vi "create config for small chassi.vi"() -> ()   [LabVIEW 2020]
uses:
  <instrlib>/_niInstr/Data Trigger/v1/Shared/Public/Edge Configuration Trigger Slope.ctl
  <vilib>/Utility/xml.llb/Write to XML File(string).vi
  <instrlib>/_niInstr/Data Trigger/v1/Shared/niInstr Data Trigger v1 Shared.lvlib
panel:
  in  "diff const [ns] 6":dbl
  in  "strob duration[ns] 5":dbl
  in  "Chans enable 6":T1={"Chan 0"=TRUE, "Chan 1"=TRUE, "Chan 2"=FALSE, "Chan 3"=FALSE, "Chan 4"=FALSE, "Chan 5"=FALSE, "Chan 6"=FALSE, "Chan 7"=FALSE}
  in  "Trapez config 6":T2={"k [ns] "=1100, "m [ns] "=200, "t_decay [ns]  "=65000, "Get energy at %\n of flat top"=70}
  in  "common trig 5172":T4={"level (V)"=-0.01, "hysteresis (V)"=0.001, "trigger slope"=enum."Negative"}
  in  "common trig 5170R 2-3":T4={"level (V)"=-0.01, "hysteresis (V)"=0.001, "trigger slope"=enum."Negative"}
  in  "common trig 5170R 0-1":T4={"level (V)"=-0.01, "hysteresis (V)"=0.001, "trigger slope"=enum."Negative"}
  in  "Enum":enum16{"Set common configs", "Write XML file"}(ring)
  in  "file name":string
  out "Writing done successfully":bool
  in  "folder":path
  in  "TAC delay":dbl
  in  "marker duration":dbl
  in  "shift marker":dbl
  in  "f":dbl
  in  "trig cfd":T4={"level (V)"=-0.01, "hysteresis (V)"=0.001, "trigger slope"=enum."Negative"}
  in  "trig marker":T4={"level (V)"=-0.01, "hysteresis (V)"=0.001, "trigger slope"=enum."Negative"}
  in  "diff const [ns] 5":dbl
  in  "BGO marker\nduration[ns] 5":dbl
  in  "Trigger Cluster 5":T5={"trig config 0"={"level (V)"=-0.01, "hysteresis (V)"=0.001, "trigger slope"=enum."Negative"}, "trig config 1"={"level (V)"=-0.01, "hysteresis (V)"=0.001, "trigger slope"=enum."Negative"}, "trig config 2"={"level (V)"=0.0, "hysteresis (V)"=0.0, "trigger slope"=enum."Positive"}, "trig config 3"={"level (V)"=0.0, "hysteresis (V)"=0.0, "trigger slope"=enum."Positive"}, "trig config 4"={"level (V)"=0.0, "hysteresis (V)"=0.0, "trigger slope"=enum."Positive"}, "trig config 5"={"level (V)"=0.0, "hysteresis (V)"=0.0, "trigger slope"=enum."Positive"}, "trig config 6"={"level (V)"=0.0, "hysteresis (V)"=0.0, "trigger slope"=enum."Positive"}, "trig config 7"={"level (V)"=0.0, "hysteresis (V)"=0.0, "trigger slope"=enum."Positive"}}
  in  "Calibr coef 5":T6={"calibr coef ch 0"={"a"=1.0, "b"=0.0}, "calibr coef ch 1"={"a"=1.0, "b"=0.0}, "calibr coef ch 2"={"a"=1.0, "b"=0.0}, "calibr coef ch 3"={"a"=1.0, "b"=0.0}, "calibr coef ch 4"={"a"=1.0, "b"=0.0}, "calibr coef ch 5"={"a"=1.0, "b"=0.0}, "calibr coef ch 6"={"a"=1.0, "b"=0.0}, "calibr coef ch 7"={"a"=1.0, "b"=0.0}}
  in  "Trapez config 5":T2={"k [ns] "=1100, "m [ns] "=200, "t_decay [ns]  "=65000, "Get energy at %\n of flat top"=70}
  in  "Chans enable 5":T1={"Chan 0"=TRUE, "Chan 1"=TRUE, "Chan 2"=FALSE, "Chan 3"=FALSE, "Chan 4"=FALSE, "Chan 5"=FALSE, "Chan 6"=FALSE, "Chan 7"=FALSE}
  in  "diff const [ns] 4":dbl
  in  "strob duration[ns] 4":dbl
  in  "Trigger Cluster 4":T5={"trig config 0"={"level (V)"=-0.01, "hysteresis (V)"=0.001, "trigger slope"=enum."Negative"}, "trig config 1"={"level (V)"=-0.01, "hysteresis (V)"=0.001, "trigger slope"=enum."Negative"}, "trig config 2"={"level (V)"=0.0, "hysteresis (V)"=0.0, "trigger slope"=enum."Positive"}, "trig config 3"={"level (V)"=0.0, "hysteresis (V)"=0.0, "trigger slope"=enum."Positive"}, "trig config 4"={"level (V)"=0.0, "hysteresis (V)"=0.0, "trigger slope"=enum."Positive"}, "trig config 5"={"level (V)"=0.0, "hysteresis (V)"=0.0, "trigger slope"=enum."Positive"}, "trig config 6"={"level (V)"=0.0, "hysteresis (V)"=0.0, "trigger slope"=enum."Positive"}, "trig config 7"={"level (V)"=0.0, "hysteresis (V)"=0.0, "trigger slope"=enum."Positive"}}
  in  "Calibr coef 4":T6={"calibr coef ch 0"={"a"=1.0, "b"=0.0}, "calibr coef ch 1"={"a"=1.0, "b"=0.0}, "calibr coef ch 2"={"a"=1.0, "b"=0.0}, "calibr coef ch 3"={"a"=1.0, "b"=0.0}, "calibr coef ch 4"={"a"=1.0, "b"=0.0}, "calibr coef ch 5"={"a"=1.0, "b"=0.0}, "calibr coef ch 6"={"a"=1.0, "b"=0.0}, "calibr coef ch 7"={"a"=1.0, "b"=0.0}}
  in  "Trapez config 4":T2={"k [ns] "=1100, "m [ns] "=200, "t_decay [ns]  "=65000, "Get energy at %\n of flat top"=70}
  in  "Chans enable 4":T1={"Chan 0"=TRUE, "Chan 1"=TRUE, "Chan 2"=FALSE, "Chan 3"=FALSE, "Chan 4"=FALSE, "Chan 5"=FALSE, "Chan 6"=FALSE, "Chan 7"=FALSE}
  in  "diff const [ns] 3":dbl
  in  "strob duration[ns] 3":dbl
  in  "Trigger Cluster 3":T5={"trig config 0"={"level (V)"=-0.01, "hysteresis (V)"=0.001, "trigger slope"=enum."Negative"}, "trig config 1"={"level (V)"=-0.01, "hysteresis (V)"=0.001, "trigger slope"=enum."Negative"}, "trig config 2"={"level (V)"=0.0, "hysteresis (V)"=0.0, "trigger slope"=enum."Positive"}, "trig config 3"={"level (V)"=0.0, "hysteresis (V)"=0.0, "trigger slope"=enum."Positive"}, "trig config 4"={"level (V)"=0.0, "hysteresis (V)"=0.0, "trigger slope"=enum."Positive"}, "trig config 5"={"level (V)"=0.0, "hysteresis (V)"=0.0, "trigger slope"=enum."Positive"}, "trig config 6"={"level (V)"=0.0, "hysteresis (V)"=0.0, "trigger slope"=enum."Positive"}, "trig config 7"={"level (V)"=0.0, "hysteresis (V)"=0.0, "trigger slope"=enum."Positive"}}
  in  "Calibr coef 3":T6={"calibr coef ch 0"={"a"=1.0, "b"=0.0}, "calibr coef ch 1"={"a"=1.0, "b"=0.0}, "calibr coef ch 2"={"a"=1.0, "b"=0.0}, "calibr coef ch 3"={"a"=1.0, "b"=0.0}, "calibr coef ch 4"={"a"=1.0, "b"=0.0}, "calibr coef ch 5"={"a"=1.0, "b"=0.0}, "calibr coef ch 6"={"a"=1.0, "b"=0.0}, "calibr coef ch 7"={"a"=1.0, "b"=0.0}}
  in  "Trapez config 3":T2={"k [ns] "=1100, "m [ns] "=200, "t_decay [ns]  "=65000, "Get energy at %\n of flat top"=70}
  in  "Chans enable 3":T1={"Chan 0"=TRUE, "Chan 1"=TRUE, "Chan 2"=FALSE, "Chan 3"=FALSE, "Chan 4"=FALSE, "Chan 5"=FALSE, "Chan 6"=FALSE, "Chan 7"=FALSE}
  in  "diff const [ns] 2":dbl
  in  "strob duration[ns] 2":dbl
  in  "Trigger Cluster 2":T5={"trig config 0"={"level (V)"=-0.01, "hysteresis (V)"=0.001, "trigger slope"=enum."Negative"}, "trig config 1"={"level (V)"=-0.01, "hysteresis (V)"=0.001, "trigger slope"=enum."Negative"}, "trig config 2"={"level (V)"=0.0, "hysteresis (V)"=0.0, "trigger slope"=enum."Positive"}, "trig config 3"={"level (V)"=0.0, "hysteresis (V)"=0.0, "trigger slope"=enum."Positive"}, "trig config 4"={"level (V)"=0.0, "hysteresis (V)"=0.0, "trigger slope"=enum."Positive"}, "trig config 5"={"level (V)"=0.0, "hysteresis (V)"=0.0, "trigger slope"=enum."Positive"}, "trig config 6"={"level (V)"=0.0, "hysteresis (V)"=0.0, "trigger slope"=enum."Positive"}, "trig config 7"={"level (V)"=0.0, "hysteresis (V)"=0.0, "trigger slope"=enum."Positive"}}
  in  "Calibr coef 2":T6={"calibr coef ch 0"={"a"=1.0, "b"=0.0}, "calibr coef ch 1"={"a"=1.0, "b"=0.0}, "calibr coef ch 2"={"a"=1.0, "b"=0.0}, "calibr coef ch 3"={"a"=1.0, "b"=0.0}, "calibr coef ch 4"={"a"=1.0, "b"=0.0}, "calibr coef ch 5"={"a"=1.0, "b"=0.0}, "calibr coef ch 6"={"a"=1.0, "b"=0.0}, "calibr coef ch 7"={"a"=1.0, "b"=0.0}}
  in  "Trapez config 2":T2={"k [ns] "=1100, "m [ns] "=200, "t_decay [ns]  "=65000, "Get energy at %\n of flat top"=70}
  in  "Chans enable 2":T1={"Chan 0"=TRUE, "Chan 1"=TRUE, "Chan 2"=FALSE, "Chan 3"=FALSE, "Chan 4"=FALSE, "Chan 5"=FALSE, "Chan 6"=FALSE, "Chan 7"=FALSE}
  in  "diff const [ns]":dbl
  in  "strob duration[ns]":dbl
  in  "Trigger Cluster":T5={"trig config 0"={"level (V)"=-0.01, "hysteresis (V)"=0.001, "trigger slope"=enum."Negative"}, "trig config 1"={"level (V)"=-0.01, "hysteresis (V)"=0.001, "trigger slope"=enum."Negative"}, "trig config 2"={"level (V)"=0.0, "hysteresis (V)"=0.0, "trigger slope"=enum."Positive"}, "trig config 3"={"level (V)"=0.0, "hysteresis (V)"=0.0, "trigger slope"=enum."Positive"}, "trig config 4"={"level (V)"=0.0, "hysteresis (V)"=0.0, "trigger slope"=enum."Positive"}, "trig config 5"={"level (V)"=0.0, "hysteresis (V)"=0.0, "trigger slope"=enum."Positive"}, "trig config 6"={"level (V)"=0.0, "hysteresis (V)"=0.0, "trigger slope"=enum."Positive"}, "trig config 7"={"level (V)"=0.0, "hysteresis (V)"=0.0, "trigger slope"=enum."Positive"}}
  in  "Calibr coef":T6={"calibr coef ch 0"={"a"=1.0, "b"=0.0}, "calibr coef ch 1"={"a"=1.0, "b"=0.0}, "calibr coef ch 2"={"a"=1.0, "b"=0.0}, "calibr coef ch 3"={"a"=1.0, "b"=0.0}, "calibr coef ch 4"={"a"=1.0, "b"=0.0}, "calibr coef ch 5"={"a"=1.0, "b"=0.0}, "calibr coef ch 6"={"a"=1.0, "b"=0.0}, "calibr coef ch 7"={"a"=1.0, "b"=0.0}}
  in  "Trapez config":T2={"k [ns] "=1100, "m [ns] "=200, "t_decay [ns]  "=65000, "Get energy at %\n of flat top"=70}
  in  "Chans enable":T1={"Chan 0"=TRUE, "Chan 1"=TRUE, "Chan 2"=FALSE, "Chan 3"=FALSE, "Chan 4"=FALSE, "Chan 5"=FALSE, "Chan 6"=FALSE, "Chan 7"=FALSE}
  # "PXIe 5170R 0"
  # "PXIe 5170R 1"
  # "PXIe 5170R 2"
  # "PXIe 5170R 3"
  # "PXIe 5172 [clover]"
  # "PXIe 5764"
  # "common configs"
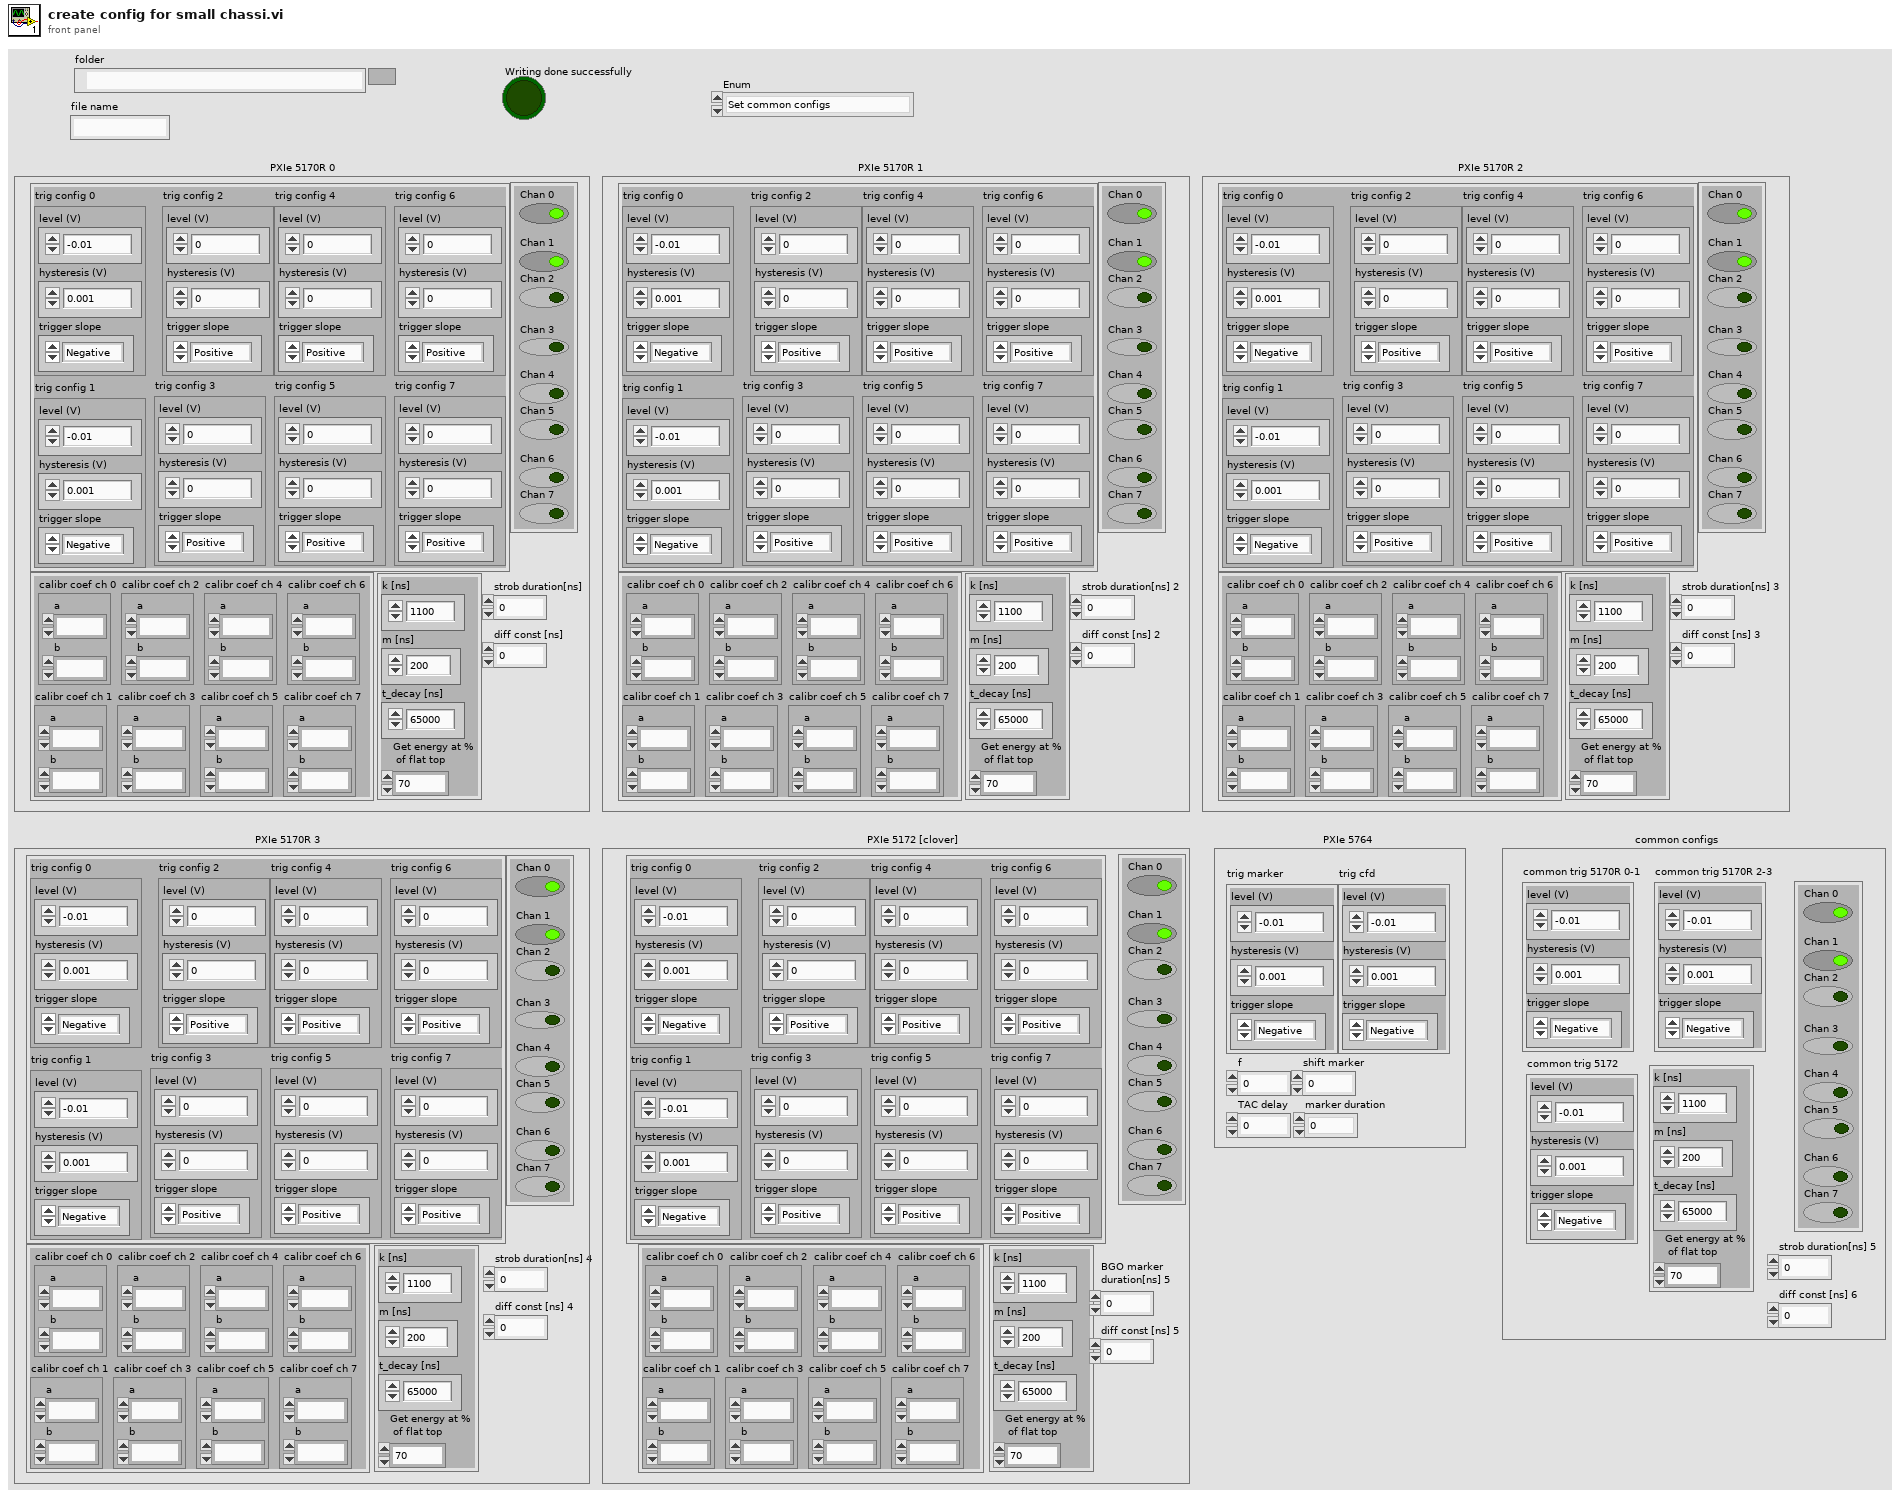
[diagram p1: front panel]
types:
  T1 = cluster{"Chan 0":bool, "Chan 1":bool, "Chan 2":bool, "Chan 3":bool, "Chan 4":bool, "Chan 5":bool, "Chan 6":bool, "Chan 7":bool}
  T2 = cluster{"k [ns] ":u16, "m [ns] ":u16, "t_decay [ns]  ":u32, "Get energy at %\n of flat top":i8}
  T3 = typedef "niInstr Data Trigger v1 Shared.lvlib/Edge Configuration Trigger Slope.ctl" = enum8{"Positive", "Negative"}
  T4 = cluster{"level (V)":dbl, "hysteresis (V)":dbl, "trigger slope":T3}
  T5 = cluster{"trig config 0":cluster{"level (V)":dbl, "hysteresis (V)":dbl, "trigger slope":T3}, "trig config 1":cluster{"level (V)":dbl, "hysteresis (V)":dbl, "trigger slope":T3}, "trig config 2":cluster{"level (V)":dbl, "hysteresis (V)":dbl, "trigger slope":T3}, "trig config 3":cluster{"level (V)":dbl, "hysteresis (V)":dbl, "trigger slope":T3}, "trig config 4":cluster{"level (V)":dbl, "hysteresis (V)":dbl, "trigger slope":T3}, "trig config 5":cluster{"level (V)":dbl, "hysteresis (V)":dbl, "trigger slope":T3}, "trig config 6":cluster{"level (V)":dbl, "hysteresis (V)":dbl, "trigger slope":T3}, "trig config 7":cluster{"level (V)":dbl, "hysteresis (V)":dbl, "trigger slope":T3}}
  T6 = cluster{"calibr coef ch 0":cluster{"a":fxp<+/-,18,9>, "b":fxp<+/-,48,24>}, "calibr coef ch 1":cluster{"a":fxp<+/-,18,9>, "b":fxp<+/-,48,24>}, "calibr coef ch 2":cluster{"a":fxp<+/-,18,9>, "b":fxp<+/-,48,24>}, "calibr coef ch 3":cluster{"a":fxp<+/-,18,9>, "b":fxp<+/-,48,24>}, "calibr coef ch 4":cluster{"a":fxp<+/-,18,9>, "b":fxp<+/-,48,24>}, "calibr coef ch 5":cluster{"a":fxp<+/-,18,9>, "b":fxp<+/-,48,24>}, "calibr coef ch 6":cluster{"a":fxp<+/-,18,9>, "b":fxp<+/-,48,24>}, "calibr coef ch 7":cluster{"a":fxp<+/-,18,9>, "b":fxp<+/-,48,24>}}
  T7 = cluster{"trig marker":cluster{"level (V)":dbl, "hysteresis (V)":dbl, "trigger slope":T3}, "trig cfd":cluster{"level (V)":dbl, "hysteresis (V)":dbl, "trigger slope":T3}, "f":dbl, "shift marker":dbl, "marker duration":dbl, "TAC delay":dbl}
  T8 = cluster{"Chans enable 5":cluster{"Chan 0":bool, "Chan 1":bool, "Chan 2":bool, "Chan 3":bool, "Chan 4":bool, "Chan 5":bool, "Chan 6":bool, "Chan 7":bool}, "Trapez config 5":cluster{"k [ns] ":u16, "m [ns] ":u16, "t_decay [ns]  ":u32, "Get energy at %\n of flat top":i8}, "Trigger Cluster 5":cluster{"trig config 0":cluster{"level (V)":dbl, "hysteresis (V)":dbl, "trigger slope":T3}, "trig config 1":cluster{"level (V)":dbl, "hysteresis (V)":dbl, "trigger slope":T3}, "trig config 2":cluster{"level (V)":dbl, "hysteresis (V)":dbl, "trigger slope":T3}, "trig config 3":cluster{"level (V)":dbl, "hysteresis (V)":dbl, "trigger slope":T3}, "trig config 4":cluster{"level (V)":dbl, "hysteresis (V)":dbl, "trigger slope":T3}, "trig config 5":cluster{"level (V)":dbl, "hysteresis (V)":dbl, "trigger slope":T3}, "trig config 6":cluster{"level (V)":dbl, "hysteresis (V)":dbl, "trigger slope":T3}, "trig config 7":cluster{"level (V)":dbl, "hysteresis (V)":dbl, "trigger slope":T3}}, "Calibr coef 5":cluster{"calibr coef ch 0":cluster{"a":fxp<+/-,18,9>, "b":fxp<+/-,48,24>}, "calibr coef ch 1":cluster{"a":fxp<+/-,18,9>, "b":fxp<+/-,48,24>}, "calibr coef ch 2":cluster{"a":fxp<+/-,18,9>, "b":fxp<+/-,48,24>}, "calibr coef ch 3":cluster{"a":fxp<+/-,18,9>, "b":fxp<+/-,48,24>}, "calibr coef ch 4":cluster{"a":fxp<+/-,18,9>, "b":fxp<+/-,48,24>}, "calibr coef ch 5":cluster{"a":fxp<+/-,18,9>, "b":fxp<+/-,48,24>}, "calibr coef ch 6":cluster{"a":fxp<+/-,18,9>, "b":fxp<+/-,48,24>}, "calibr coef ch 7":cluster{"a":fxp<+/-,18,9>, "b":fxp<+/-,48,24>}}, "BGO marker\nduration[ns] 5":dbl, "diff const [ns] 5":dbl}
  T9 = cluster{"5170R 0":cluster{"Chans enable":cluster{"Chan 0":bool, "Chan 1":bool, "Chan 2":bool, "Chan 3":bool, "Chan 4":bool, "Chan 5":bool, "Chan 6":bool, "Chan 7":bool}, "Trapez config":cluster{"k [ns] ":u16, "m [ns] ":u16, "t_decay [ns]  ":u32, "Get energy at %\n of flat top":i8}, "Trigger Cluster":cluster{"trig config 0":cluster{"level (V)":dbl, "hysteresis (V)":dbl, "trigger slope":T3}, "trig config 1":cluster{"level (V)":dbl, "hysteresis (V)":dbl, "trigger slope":T3}, "trig config 2":cluster{"level (V)":dbl, "hysteresis (V)":dbl, "trigger slope":T3}, "trig config 3":cluster{"level (V)":dbl, "hysteresis (V)":dbl, "trigger slope":T3}, "trig config 4":cluster{"level (V)":dbl, "hysteresis (V)":dbl, "trigger slope":T3}, "trig config 5":cluster{"level (V)":dbl, "hysteresis (V)":dbl, "trigger slope":T3}, "trig config 6":cluster{"level (V)":dbl, "hysteresis (V)":dbl, "trigger slope":T3}, "trig config 7":cluster{"level (V)":dbl, "hysteresis (V)":dbl, "trigger slope":T3}}, "Calibr coef":cluster{"calibr coef ch 0":cluster{"a":fxp<+/-,18,9>, "b":fxp<+/-,48,24>}, "calibr coef ch 1":cluster{"a":fxp<+/-,18,9>, "b":fxp<+/-,48,24>}, "calibr coef ch 2":cluster{"a":fxp<+/-,18,9>, "b":fxp<+/-,48,24>}, "calibr coef ch 3":cluster{"a":fxp<+/-,18,9>, "b":fxp<+/-,48,24>}, "calibr coef ch 4":cluster{"a":fxp<+/-,18,9>, "b":fxp<+/-,48,24>}, "calibr coef ch 5":cluster{"a":fxp<+/-,18,9>, "b":fxp<+/-,48,24>}, "calibr coef ch 6":cluster{"a":fxp<+/-,18,9>, "b":fxp<+/-,48,24>}, "calibr coef ch 7":cluster{"a":fxp<+/-,18,9>, "b":fxp<+/-,48,24>}}, "strob duration[ns]":dbl, "diff const [ns]":dbl}, "5170R 1":cluster{"Chans enable":cluster{"Chan 0":bool, "Chan 1":bool, "Chan 2":bool, "Chan 3":bool, "Chan 4":bool, "Chan 5":bool, "Chan 6":bool, "Chan 7":bool}, "Trapez config":cluster{"k [ns] ":u16, "m [ns] ":u16, "t_decay [ns]  ":u32, "Get energy at %\n of flat top":i8}, "Trigger Cluster":cluster{"trig config 0":cluster{"level (V)":dbl, "hysteresis (V)":dbl, "trigger slope":T3}, "trig config 1":cluster{"level (V)":dbl, "hysteresis (V)":dbl, "trigger slope":T3}, "trig config 2":cluster{"level (V)":dbl, "hysteresis (V)":dbl, "trigger slope":T3}, "trig config 3":cluster{"level (V)":dbl, "hysteresis (V)":dbl, "trigger slope":T3}, "trig config 4":cluster{"level (V)":dbl, "hysteresis (V)":dbl, "trigger slope":T3}, "trig config 5":cluster{"level (V)":dbl, "hysteresis (V)":dbl, "trigger slope":T3}, "trig config 6":cluster{"level (V)":dbl, "hysteresis (V)":dbl, "trigger slope":T3}, "trig config 7":cluster{"level (V)":dbl, "hysteresis (V)":dbl, "trigger slope":T3}}, "Calibr coef":cluster{"calibr coef ch 0":cluster{"a":fxp<+/-,18,9>, "b":fxp<+/-,48,24>}, "calibr coef ch 1":cluster{"a":fxp<+/-,18,9>, "b":fxp<+/-,48,24>}, "calibr coef ch 2":cluster{"a":fxp<+/-,18,9>, "b":fxp<+/-,48,24>}, "calibr coef ch 3":cluster{"a":fxp<+/-,18,9>, "b":fxp<+/-,48,24>}, "calibr coef ch 4":cluster{"a":fxp<+/-,18,9>, "b":fxp<+/-,48,24>}, "calibr coef ch 5":cluster{"a":fxp<+/-,18,9>, "b":fxp<+/-,48,24>}, "calibr coef ch 6":cluster{"a":fxp<+/-,18,9>, "b":fxp<+/-,48,24>}, "calibr coef ch 7":cluster{"a":fxp<+/-,18,9>, "b":fxp<+/-,48,24>}}, "strob duration[ns]":dbl, "diff const [ns]":dbl}, "5170R 2":cluster{"Chans enable":cluster{"Chan 0":bool, "Chan 1":bool, "Chan 2":bool, "Chan 3":bool, "Chan 4":bool, "Chan 5":bool, "Chan 6":bool, "Chan 7":bool}, "Trapez config":cluster{"k [ns] ":u16, "m [ns] ":u16, "t_decay [ns]  ":u32, "Get energy at %\n of flat top":i8}, "Trigger Cluster":cluster{"trig config 0":cluster{"level (V)":dbl, "hysteresis (V)":dbl, "trigger slope":T3}, "trig config 1":cluster{"level (V)":dbl, "hysteresis (V)":dbl, "trigger slope":T3}, "trig config 2":cluster{"level (V)":dbl, "hysteresis (V)":dbl, "trigger slope":T3}, "trig config 3":cluster{"level (V)":dbl, "hysteresis (V)":dbl, "trigger slope":T3}, "trig config 4":cluster{"level (V)":dbl, "hysteresis (V)":dbl, "trigger slope":T3}, "trig config 5":cluster{"level (V)":dbl, "hysteresis (V)":dbl, "trigger slope":T3}, "trig config 6":cluster{"level (V)":dbl, "hysteresis (V)":dbl, "trigger slope":T3}, "trig config 7":cluster{"level (V)":dbl, "hysteresis (V)":dbl, "trigger slope":T3}}, "Calibr coef":cluster{"calibr coef ch 0":cluster{"a":fxp<+/-,18,9>, "b":fxp<+/-,48,24>}, "calibr coef ch 1":cluster{"a":fxp<+/-,18,9>, "b":fxp<+/-,48,24>}, "calibr coef ch 2":cluster{"a":fxp<+/-,18,9>, "b":fxp<+/-,48,24>}, "calibr coef ch 3":cluster{"a":fxp<+/-,18,9>, "b":fxp<+/-,48,24>}, "calibr coef ch 4":cluster{"a":fxp<+/-,18,9>, "b":fxp<+/-,48,24>}, "calibr coef ch 5":cluster{"a":fxp<+/-,18,9>, "b":fxp<+/-,48,24>}, "calibr coef ch 6":cluster{"a":fxp<+/-,18,9>, "b":fxp<+/-,48,24>}, "calibr coef ch 7":cluster{"a":fxp<+/-,18,9>, "b":fxp<+/-,48,24>}}, "strob duration[ns]":dbl, "diff const [ns]":dbl}, "5170R 3":cluster{"Chans enable":cluster{"Chan 0":bool, "Chan 1":bool, "Chan 2":bool, "Chan 3":bool, "Chan 4":bool, "Chan 5":bool, "Chan 6":bool, "Chan 7":bool}, "Trapez config":cluster{"k [ns] ":u16, "m [ns] ":u16, "t_decay [ns]  ":u32, "Get energy at %\n of flat top":i8}, "Trigger Cluster":cluster{"trig config 0":cluster{"level (V)":dbl, "hysteresis (V)":dbl, "trigger slope":T3}, "trig config 1":cluster{"level (V)":dbl, "hysteresis (V)":dbl, "trigger slope":T3}, "trig config 2":cluster{"level (V)":dbl, "hysteresis (V)":dbl, "trigger slope":T3}, "trig config 3":cluster{"level (V)":dbl, "hysteresis (V)":dbl, "trigger slope":T3}, "trig config 4":cluster{"level (V)":dbl, "hysteresis (V)":dbl, "trigger slope":T3}, "trig config 5":cluster{"level (V)":dbl, "hysteresis (V)":dbl, "trigger slope":T3}, "trig config 6":cluster{"level (V)":dbl, "hysteresis (V)":dbl, "trigger slope":T3}, "trig config 7":cluster{"level (V)":dbl, "hysteresis (V)":dbl, "trigger slope":T3}}, "Calibr coef":cluster{"calibr coef ch 0":cluster{"a":fxp<+/-,18,9>, "b":fxp<+/-,48,24>}, "calibr coef ch 1":cluster{"a":fxp<+/-,18,9>, "b":fxp<+/-,48,24>}, "calibr coef ch 2":cluster{"a":fxp<+/-,18,9>, "b":fxp<+/-,48,24>}, "calibr coef ch 3":cluster{"a":fxp<+/-,18,9>, "b":fxp<+/-,48,24>}, "calibr coef ch 4":cluster{"a":fxp<+/-,18,9>, "b":fxp<+/-,48,24>}, "calibr coef ch 5":cluster{"a":fxp<+/-,18,9>, "b":fxp<+/-,48,24>}, "calibr coef ch 6":cluster{"a":fxp<+/-,18,9>, "b":fxp<+/-,48,24>}, "calibr coef ch 7":cluster{"a":fxp<+/-,18,9>, "b":fxp<+/-,48,24>}}, "strob duration[ns]":dbl, "diff const [ns]":dbl}, "5172":cluster{"Chans enable 5":cluster{"Chan 0":bool, "Chan 1":bool, "Chan 2":bool, "Chan 3":bool, "Chan 4":bool, "Chan 5":bool, "Chan 6":bool, "Chan 7":bool}, "Trapez config 5":cluster{"k [ns] ":u16, "m [ns] ":u16, "t_decay [ns]  ":u32, "Get energy at %\n of flat top":i8}, "Trigger Cluster 5":cluster{"trig config 0":cluster{"level (V)":dbl, "hysteresis (V)":dbl, "trigger slope":T3}, "trig config 1":cluster{"level (V)":dbl, "hysteresis (V)":dbl, "trigger slope":T3}, "trig config 2":cluster{"level (V)":dbl, "hysteresis (V)":dbl, "trigger slope":T3}, "trig config 3":cluster{"level (V)":dbl, "hysteresis (V)":dbl, "trigger slope":T3}, "trig config 4":cluster{"level (V)":dbl, "hysteresis (V)":dbl, "trigger slope":T3}, "trig config 5":cluster{"level (V)":dbl, "hysteresis (V)":dbl, "trigger slope":T3}, "trig config 6":cluster{"level (V)":dbl, "hysteresis (V)":dbl, "trigger slope":T3}, "trig config 7":cluster{"level (V)":dbl, "hysteresis (V)":dbl, "trigger slope":T3}}, "Calibr coef 5":cluster{"calibr coef ch 0":cluster{"a":fxp<+/-,18,9>, "b":fxp<+/-,48,24>}, "calibr coef ch 1":cluster{"a":fxp<+/-,18,9>, "b":fxp<+/-,48,24>}, "calibr coef ch 2":cluster{"a":fxp<+/-,18,9>, "b":fxp<+/-,48,24>}, "calibr coef ch 3":cluster{"a":fxp<+/-,18,9>, "b":fxp<+/-,48,24>}, "calibr coef ch 4":cluster{"a":fxp<+/-,18,9>, "b":fxp<+/-,48,24>}, "calibr coef ch 5":cluster{"a":fxp<+/-,18,9>, "b":fxp<+/-,48,24>}, "calibr coef ch 6":cluster{"a":fxp<+/-,18,9>, "b":fxp<+/-,48,24>}, "calibr coef ch 7":cluster{"a":fxp<+/-,18,9>, "b":fxp<+/-,48,24>}}, "BGO marker\nduration[ns] 5":dbl, "diff const [ns] 5":dbl}, "5764":cluster{"trig marker":cluster{"level (V)":dbl, "hysteresis (V)":dbl, "trigger slope":T3}, "trig cfd":cluster{"level (V)":dbl, "hysteresis (V)":dbl, "trigger slope":T3}, "f":dbl, "shift marker":dbl, "marker duration":dbl, "TAC delay":dbl}}
  T10 = cluster{"Chans enable":cluster{"Chan 0":bool, "Chan 1":bool, "Chan 2":bool, "Chan 3":bool, "Chan 4":bool, "Chan 5":bool, "Chan 6":bool, "Chan 7":bool}, "Trapez config":cluster{"k [ns] ":u16, "m [ns] ":u16, "t_decay [ns]  ":u32, "Get energy at %\n of flat top":i8}, "Trigger Cluster":cluster{"trig config 0":cluster{"level (V)":dbl, "hysteresis (V)":dbl, "trigger slope":T3}, "trig config 1":cluster{"level (V)":dbl, "hysteresis (V)":dbl, "trigger slope":T3}, "trig config 2":cluster{"level (V)":dbl, "hysteresis (V)":dbl, "trigger slope":T3}, "trig config 3":cluster{"level (V)":dbl, "hysteresis (V)":dbl, "trigger slope":T3}, "trig config 4":cluster{"level (V)":dbl, "hysteresis (V)":dbl, "trigger slope":T3}, "trig config 5":cluster{"level (V)":dbl, "hysteresis (V)":dbl, "trigger slope":T3}, "trig config 6":cluster{"level (V)":dbl, "hysteresis (V)":dbl, "trigger slope":T3}, "trig config 7":cluster{"level (V)":dbl, "hysteresis (V)":dbl, "trigger slope":T3}}, "Calibr coef":cluster{"calibr coef ch 0":cluster{"a":fxp<+/-,18,9>, "b":fxp<+/-,48,24>}, "calibr coef ch 1":cluster{"a":fxp<+/-,18,9>, "b":fxp<+/-,48,24>}, "calibr coef ch 2":cluster{"a":fxp<+/-,18,9>, "b":fxp<+/-,48,24>}, "calibr coef ch 3":cluster{"a":fxp<+/-,18,9>, "b":fxp<+/-,48,24>}, "calibr coef ch 4":cluster{"a":fxp<+/-,18,9>, "b":fxp<+/-,48,24>}, "calibr coef ch 5":cluster{"a":fxp<+/-,18,9>, "b":fxp<+/-,48,24>}, "calibr coef ch 6":cluster{"a":fxp<+/-,18,9>, "b":fxp<+/-,48,24>}, "calibr coef ch 7":cluster{"a":fxp<+/-,18,9>, "b":fxp<+/-,48,24>}}, "strob duration[ns]":dbl, "diff const [ns]":dbl}
  T11 = cluster{"Chassi 0":cluster{"5170R 0":cluster{"Chans enable":cluster{"Chan 0":bool, "Chan 1":bool, "Chan 2":bool, "Chan 3":bool, "Chan 4":bool, "Chan 5":bool, "Chan 6":bool, "Chan 7":bool}, "Trapez config":cluster{"k [ns] ":u16, "m [ns] ":u16, "t_decay [ns]  ":u32, "Get energy at %\n of flat top":i8}, "Trigger Cluster":cluster{"trig config 0":cluster{"level (V)":dbl, "hysteresis (V)":dbl, "trigger slope":T3}, "trig config 1":cluster{"level (V)":dbl, "hysteresis (V)":dbl, "trigger slope":T3}, "trig config 2":cluster{"level (V)":dbl, "hysteresis (V)":dbl, "trigger slope":T3}, "trig config 3":cluster{"level (V)":dbl, "hysteresis (V)":dbl, "trigger slope":T3}, "trig config 4":cluster{"level (V)":dbl, "hysteresis (V)":dbl, "trigger slope":T3}, "trig config 5":cluster{"level (V)":dbl, "hysteresis (V)":dbl, "trigger slope":T3}, "trig config 6":cluster{"level (V)":dbl, "hysteresis (V)":dbl, "trigger slope":T3}, "trig config 7":cluster{"level (V)":dbl, "hysteresis (V)":dbl, "trigger slope":T3}}, "Calibr coef":cluster{"calibr coef ch 0":cluster{"a":fxp<+/-,18,9>, "b":fxp<+/-,48,24>}, "calibr coef ch 1":cluster{"a":fxp<+/-,18,9>, "b":fxp<+/-,48,24>}, "calibr coef ch 2":cluster{"a":fxp<+/-,18,9>, "b":fxp<+/-,48,24>}, "calibr coef ch 3":cluster{"a":fxp<+/-,18,9>, "b":fxp<+/-,48,24>}, "calibr coef ch 4":cluster{"a":fxp<+/-,18,9>, "b":fxp<+/-,48,24>}, "calibr coef ch 5":cluster{"a":fxp<+/-,18,9>, "b":fxp<+/-,48,24>}, "calibr coef ch 6":cluster{"a":fxp<+/-,18,9>, "b":fxp<+/-,48,24>}, "calibr coef ch 7":cluster{"a":fxp<+/-,18,9>, "b":fxp<+/-,48,24>}}, "strob duration[ns]":dbl, "diff const [ns]":dbl}, "5170R 1":cluster{"Chans enable":cluster{"Chan 0":bool, "Chan 1":bool, "Chan 2":bool, "Chan 3":bool, "Chan 4":bool, "Chan 5":bool, "Chan 6":bool, "Chan 7":bool}, "Trapez config":cluster{"k [ns] ":u16, "m [ns] ":u16, "t_decay [ns]  ":u32, "Get energy at %\n of flat top":i8}, "Trigger Cluster":cluster{"trig config 0":cluster{"level (V)":dbl, "hysteresis (V)":dbl, "trigger slope":T3}, "trig config 1":cluster{"level (V)":dbl, "hysteresis (V)":dbl, "trigger slope":T3}, "trig config 2":cluster{"level (V)":dbl, "hysteresis (V)":dbl, "trigger slope":T3}, "trig config 3":cluster{"level (V)":dbl, "hysteresis (V)":dbl, "trigger slope":T3}, "trig config 4":cluster{"level (V)":dbl, "hysteresis (V)":dbl, "trigger slope":T3}, "trig config 5":cluster{"level (V)":dbl, "hysteresis (V)":dbl, "trigger slope":T3}, "trig config 6":cluster{"level (V)":dbl, "hysteresis (V)":dbl, "trigger slope":T3}, "trig config 7":cluster{"level (V)":dbl, "hysteresis (V)":dbl, "trigger slope":T3}}, "Calibr coef":cluster{"calibr coef ch 0":cluster{"a":fxp<+/-,18,9>, "b":fxp<+/-,48,24>}, "calibr coef ch 1":cluster{"a":fxp<+/-,18,9>, "b":fxp<+/-,48,24>}, "calibr coef ch 2":cluster{"a":fxp<+/-,18,9>, "b":fxp<+/-,48,24>}, "calibr coef ch 3":cluster{"a":fxp<+/-,18,9>, "b":fxp<+/-,48,24>}, "calibr coef ch 4":cluster{"a":fxp<+/-,18,9>, "b":fxp<+/-,48,24>}, "calibr coef ch 5":cluster{"a":fxp<+/-,18,9>, "b":fxp<+/-,48,24>}, "calibr coef ch 6":cluster{"a":fxp<+/-,18,9>, "b":fxp<+/-,48,24>}, "calibr coef ch 7":cluster{"a":fxp<+/-,18,9>, "b":fxp<+/-,48,24>}}, "strob duration[ns]":dbl, "diff const [ns]":dbl}, "5170R 2":cluster{"Chans enable":cluster{"Chan 0":bool, "Chan 1":bool, "Chan 2":bool, "Chan 3":bool, "Chan 4":bool, "Chan 5":bool, "Chan 6":bool, "Chan 7":bool}, "Trapez config":cluster{"k [ns] ":u16, "m [ns] ":u16, "t_decay [ns]  ":u32, "Get energy at %\n of flat top":i8}, "Trigger Cluster":cluster{"trig config 0":cluster{"level (V)":dbl, "hysteresis (V)":dbl, "trigger slope":T3}, "trig config 1":cluster{"level (V)":dbl, "hysteresis (V)":dbl, "trigger slope":T3}, "trig config 2":cluster{"level (V)":dbl, "hysteresis (V)":dbl, "trigger slope":T3}, "trig config 3":cluster{"level (V)":dbl, "hysteresis (V)":dbl, "trigger slope":T3}, "trig config 4":cluster{"level (V)":dbl, "hysteresis (V)":dbl, "trigger slope":T3}, "trig config 5":cluster{"level (V)":dbl, "hysteresis (V)":dbl, "trigger slope":T3}, "trig config 6":cluster{"level (V)":dbl, "hysteresis (V)":dbl, "trigger slope":T3}, "trig config 7":cluster{"level (V)":dbl, "hysteresis (V)":dbl, "trigger slope":T3}}, "Calibr coef":cluster{"calibr coef ch 0":cluster{"a":fxp<+/-,18,9>, "b":fxp<+/-,48,24>}, "calibr coef ch 1":cluster{"a":fxp<+/-,18,9>, "b":fxp<+/-,48,24>}, "calibr coef ch 2":cluster{"a":fxp<+/-,18,9>, "b":fxp<+/-,48,24>}, "calibr coef ch 3":cluster{"a":fxp<+/-,18,9>, "b":fxp<+/-,48,24>}, "calibr coef ch 4":cluster{"a":fxp<+/-,18,9>, "b":fxp<+/-,48,24>}, "calibr coef ch 5":cluster{"a":fxp<+/-,18,9>, "b":fxp<+/-,48,24>}, "calibr coef ch 6":cluster{"a":fxp<+/-,18,9>, "b":fxp<+/-,48,24>}, "calibr coef ch 7":cluster{"a":fxp<+/-,18,9>, "b":fxp<+/-,48,24>}}, "strob duration[ns]":dbl, "diff const [ns]":dbl}, "5170R 3":cluster{"Chans enable":cluster{"Chan 0":bool, "Chan 1":bool, "Chan 2":bool, "Chan 3":bool, "Chan 4":bool, "Chan 5":bool, "Chan 6":bool, "Chan 7":bool}, "Trapez config":cluster{"k [ns] ":u16, "m [ns] ":u16, "t_decay [ns]  ":u32, "Get energy at %\n of flat top":i8}, "Trigger Cluster":cluster{"trig config 0":cluster{"level (V)":dbl, "hysteresis (V)":dbl, "trigger slope":T3}, "trig config 1":cluster{"level (V)":dbl, "hysteresis (V)":dbl, "trigger slope":T3}, "trig config 2":cluster{"level (V)":dbl, "hysteresis (V)":dbl, "trigger slope":T3}, "trig config 3":cluster{"level (V)":dbl, "hysteresis (V)":dbl, "trigger slope":T3}, "trig config 4":cluster{"level (V)":dbl, "hysteresis (V)":dbl, "trigger slope":T3}, "trig config 5":cluster{"level (V)":dbl, "hysteresis (V)":dbl, "trigger slope":T3}, "trig config 6":cluster{"level (V)":dbl, "hysteresis (V)":dbl, "trigger slope":T3}, "trig config 7":cluster{"level (V)":dbl, "hysteresis (V)":dbl, "trigger slope":T3}}, "Calibr coef":cluster{"calibr coef ch 0":cluster{"a":fxp<+/-,18,9>, "b":fxp<+/-,48,24>}, "calibr coef ch 1":cluster{"a":fxp<+/-,18,9>, "b":fxp<+/-,48,24>}, "calibr coef ch 2":cluster{"a":fxp<+/-,18,9>, "b":fxp<+/-,48,24>}, "calibr coef ch 3":cluster{"a":fxp<+/-,18,9>, "b":fxp<+/-,48,24>}, "calibr coef ch 4":cluster{"a":fxp<+/-,18,9>, "b":fxp<+/-,48,24>}, "calibr coef ch 5":cluster{"a":fxp<+/-,18,9>, "b":fxp<+/-,48,24>}, "calibr coef ch 6":cluster{"a":fxp<+/-,18,9>, "b":fxp<+/-,48,24>}, "calibr coef ch 7":cluster{"a":fxp<+/-,18,9>, "b":fxp<+/-,48,24>}}, "strob duration[ns]":dbl, "diff const [ns]":dbl}, "5172":cluster{"Chans enable 5":cluster{"Chan 0":bool, "Chan 1":bool, "Chan 2":bool, "Chan 3":bool, "Chan 4":bool, "Chan 5":bool, "Chan 6":bool, "Chan 7":bool}, "Trapez config 5":cluster{"k [ns] ":u16, "m [ns] ":u16, "t_decay [ns]  ":u32, "Get energy at %\n of flat top":i8}, "Trigger Cluster 5":cluster{"trig config 0":cluster{"level (V)":dbl, "hysteresis (V)":dbl, "trigger slope":T3}, "trig config 1":cluster{"level (V)":dbl, "hysteresis (V)":dbl, "trigger slope":T3}, "trig config 2":cluster{"level (V)":dbl, "hysteresis (V)":dbl, "trigger slope":T3}, "trig config 3":cluster{"level (V)":dbl, "hysteresis (V)":dbl, "trigger slope":T3}, "trig config 4":cluster{"level (V)":dbl, "hysteresis (V)":dbl, "trigger slope":T3}, "trig config 5":cluster{"level (V)":dbl, "hysteresis (V)":dbl, "trigger slope":T3}, "trig config 6":cluster{"level (V)":dbl, "hysteresis (V)":dbl, "trigger slope":T3}, "trig config 7":cluster{"level (V)":dbl, "hysteresis (V)":dbl, "trigger slope":T3}}, "Calibr coef 5":cluster{"calibr coef ch 0":cluster{"a":fxp<+/-,18,9>, "b":fxp<+/-,48,24>}, "calibr coef ch 1":cluster{"a":fxp<+/-,18,9>, "b":fxp<+/-,48,24>}, "calibr coef ch 2":cluster{"a":fxp<+/-,18,9>, "b":fxp<+/-,48,24>}, "calibr coef ch 3":cluster{"a":fxp<+/-,18,9>, "b":fxp<+/-,48,24>}, "calibr coef ch 4":cluster{"a":fxp<+/-,18,9>, "b":fxp<+/-,48,24>}, "calibr coef ch 5":cluster{"a":fxp<+/-,18,9>, "b":fxp<+/-,48,24>}, "calibr coef ch 6":cluster{"a":fxp<+/-,18,9>, "b":fxp<+/-,48,24>}, "calibr coef ch 7":cluster{"a":fxp<+/-,18,9>, "b":fxp<+/-,48,24>}}, "BGO marker\nduration[ns] 5":dbl, "diff const [ns] 5":dbl}, "5764":cluster{"trig marker":cluster{"level (V)":dbl, "hysteresis (V)":dbl, "trigger slope":T3}, "trig cfd":cluster{"level (V)":dbl, "hysteresis (V)":dbl, "trigger slope":T3}, "f":dbl, "shift marker":dbl, "marker duration":dbl, "TAC delay":dbl}}}
  T12 = cluster{"common trig 5170R 0-1":cluster{"level (V)":dbl, "hysteresis (V)":dbl, "trigger slope":T3}, "common trig 5170R 0-1":cluster{"level (V)":dbl, "hysteresis (V)":dbl, "trigger slope":T3}, "common trig 5170R 0-1":cluster{"level (V)":dbl, "hysteresis (V)":dbl, "trigger slope":T3}, "common trig 5170R 0-1":cluster{"level (V)":dbl, "hysteresis (V)":dbl, "trigger slope":T3}, "common trig 5170R 0-1":cluster{"level (V)":dbl, "hysteresis (V)":dbl, "trigger slope":T3}, "common trig 5170R 0-1":cluster{"level (V)":dbl, "hysteresis (V)":dbl, "trigger slope":T3}, "common trig 5170R 0-1":cluster{"level (V)":dbl, "hysteresis (V)":dbl, "trigger slope":T3}, "common trig 5170R 0-1":cluster{"level (V)":dbl, "hysteresis (V)":dbl, "trigger slope":T3}}
  T13 = cluster{"common trig 5170R 2-3":cluster{"level (V)":dbl, "hysteresis (V)":dbl, "trigger slope":T3}, "common trig 5170R 2-3":cluster{"level (V)":dbl, "hysteresis (V)":dbl, "trigger slope":T3}, "common trig 5170R 2-3":cluster{"level (V)":dbl, "hysteresis (V)":dbl, "trigger slope":T3}, "common trig 5170R 2-3":cluster{"level (V)":dbl, "hysteresis (V)":dbl, "trigger slope":T3}, "common trig 5170R 2-3":cluster{"level (V)":dbl, "hysteresis (V)":dbl, "trigger slope":T3}, "common trig 5170R 2-3":cluster{"level (V)":dbl, "hysteresis (V)":dbl, "trigger slope":T3}, "common trig 5170R 2-3":cluster{"level (V)":dbl, "hysteresis (V)":dbl, "trigger slope":T3}, "common trig 5170R 2-3":cluster{"level (V)":dbl, "hysteresis (V)":dbl, "trigger slope":T3}}
  T14 = cluster{"common trig 5172":cluster{"level (V)":dbl, "hysteresis (V)":dbl, "trigger slope":T3}, "common trig 5172":cluster{"level (V)":dbl, "hysteresis (V)":dbl, "trigger slope":T3}, "common trig 5172":cluster{"level (V)":dbl, "hysteresis (V)":dbl, "trigger slope":T3}, "common trig 5172":cluster{"level (V)":dbl, "hysteresis (V)":dbl, "trigger slope":T3}, "common trig 5172":cluster{"level (V)":dbl, "hysteresis (V)":dbl, "trigger slope":T3}, "common trig 5172":cluster{"level (V)":dbl, "hysteresis (V)":dbl, "trigger slope":T3}, "common trig 5172":cluster{"level (V)":dbl, "hysteresis (V)":dbl, "trigger slope":T3}, "common trig 5172":cluster{"level (V)":dbl, "hysteresis (V)":dbl, "trigger slope":T3}}
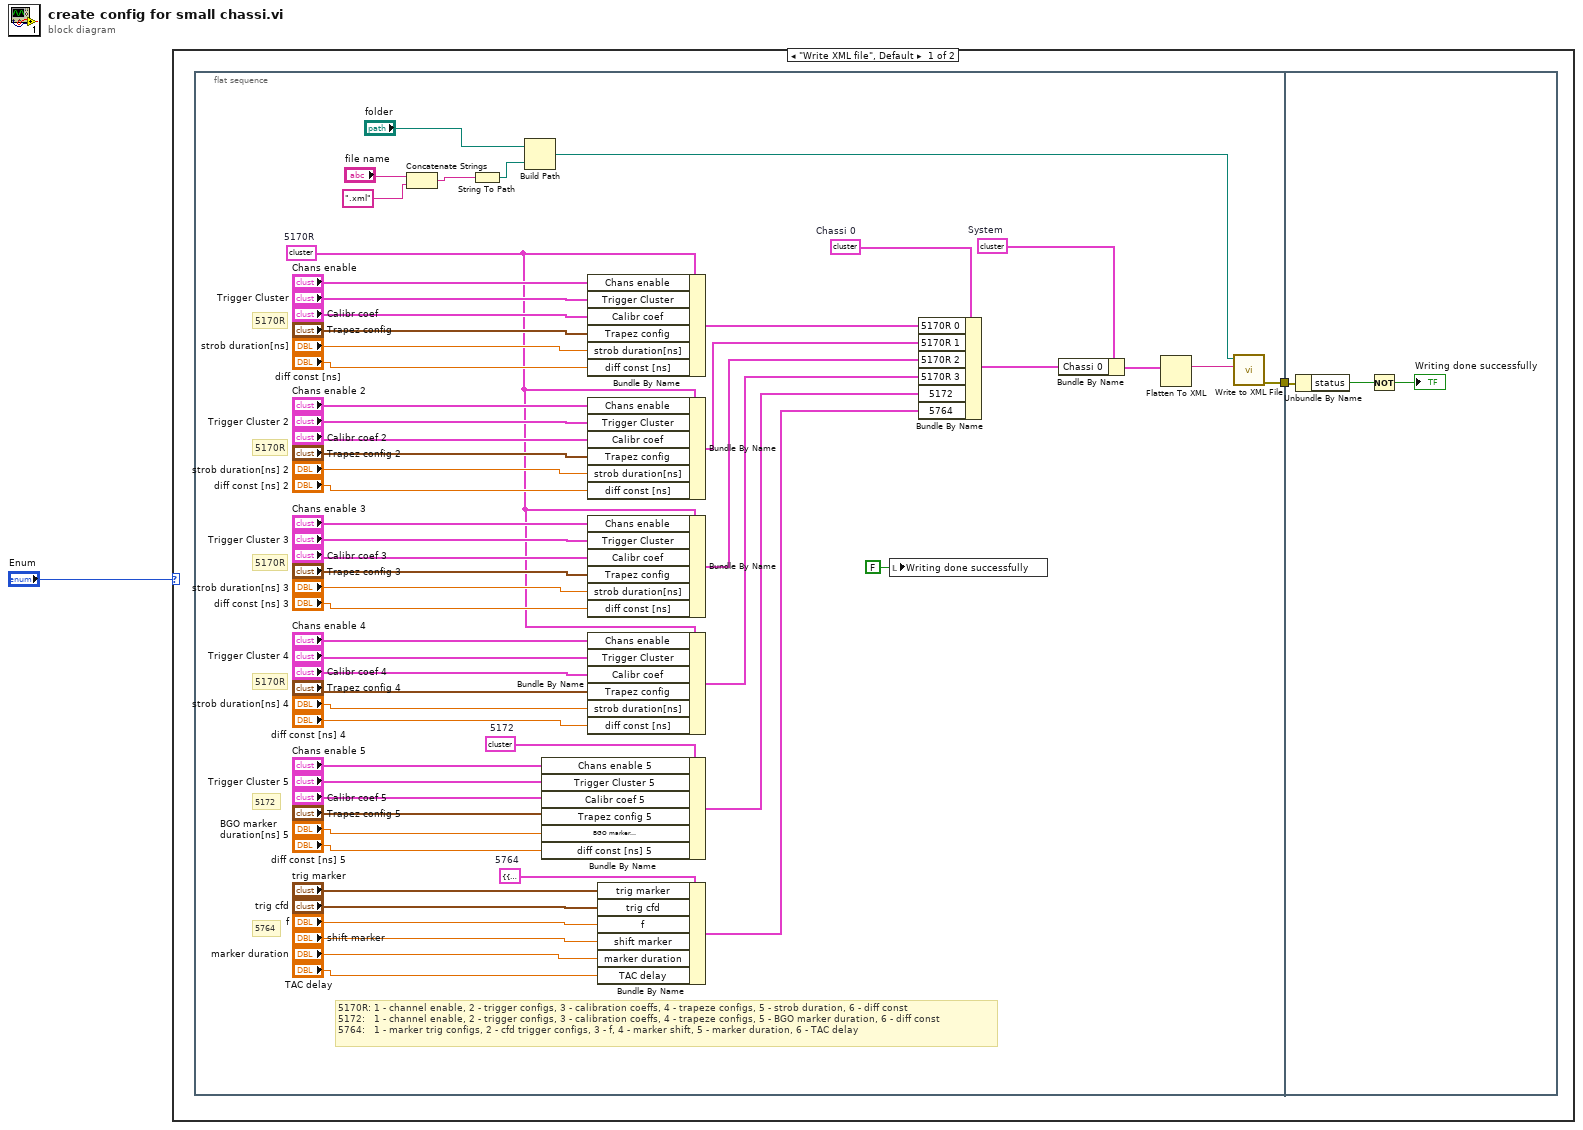
[diagram p0: block diagram]
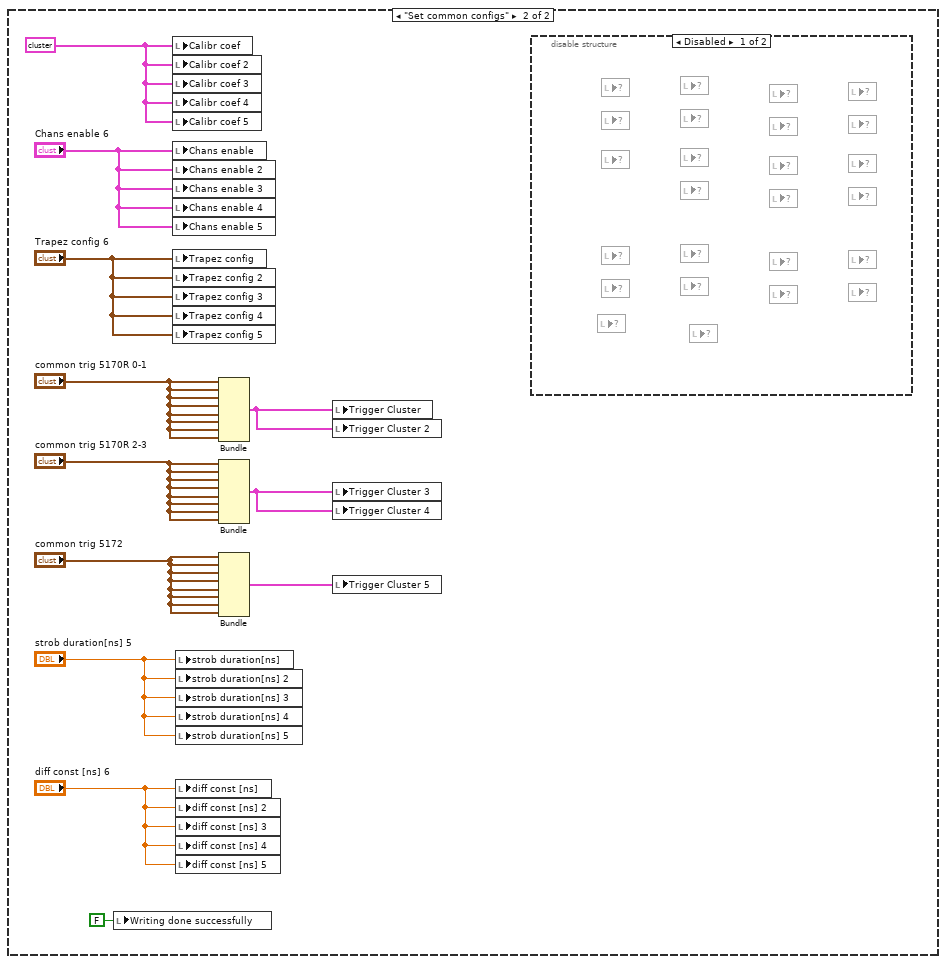
[diagram p2: hidden frame]
diagram:
  n1 = case shown="\"Write XML file\", Default" "Enum" {
    frame "Write XML file", Default {
      n2 = flat-sequence {
        tunnel: [w8] -> w2
        tunnel: w2 -> [w63]
        frame #0 {
          w28 = T7 {"trig marker"={"level (V)"=-0.01, "hysteresis (V)"=0.001, "trigger slope"=enum."Negative"}, "trig cfd"={"level (V)"=-0.01, "hysteresis (V)"=0.001, "trigger slope"=enum."Negative"}, "f"=0.0, "shift marker"=0.0, "marker duration"=0.0, "TAC delay"=0.0}  # 5764
          w35 = T8 {"Chans enable 5"={"Chan 0"=TRUE, "Chan 1"=TRUE, "Chan 2"=TRUE, "Chan 3"=TRUE, "Chan 4"=TRUE, "Chan 5"=TRUE, "Chan 6"=TRUE, "Chan 7"=TRUE}, "Trapez config 5"={"k [ns] "=1100, "m [ns] "=200, "t_decay [ns]  "=65000, "Get energy at %\n of flat top"=70}, "Trigger Cluster 5"={"trig config 0"={"level (V)"=-0.01, "hysteresis (V)"=0.001, "trigger slope"=enum."Negative"}, "trig config 1"={"level (V)"=-0.01, "hysteresis (V)"=0.001, "trigger slope"=enum."Negative"}, "trig config 2"={"level (V)"=-0.01, "hysteresis (V)"=0.001, "trigger slope"=enum."Negative"}, "trig config 3"={"level (V)"=-0.01, "hysteresis (V)"=0.001, "trigger slope"=enum."Negative"}, "trig config 4"={"level (V)"=-0.01, "hysteresis (V)"=0.001, "trigger slope"=enum."Negative"}, "trig config 5"={"level (V)"=-0.01, "hysteresis (V)"=0.001, "trigger slope"=enum."Negative"}, "trig config 6"={"level (V)"=-0.01, "hysteresis (V)"=0.001, "trigger slope"=enum."Negative"}, "trig config 7"={"level (V)"=-0.01, "hysteresis (V)"=0.001, "trigger slope"=enum."Negative"}}, "Calibr coef 5"={"calibr coef ch 0"={"a"=1.0, "b"=0.0}, "calibr coef ch 1"={"a"=1.0, "b"=0.0}, "calibr coef ch 2"={"a"=1.0, "b"=0.0}, "calibr coef ch 3"={"a"=1.0, "b"=0.0}, "calibr coef ch 4"={"a"=1.0, "b"=0.0}, "calibr coef ch 5"={"a"=1.0, "b"=0.0}, "calibr coef ch 6"={"a"=1.0, "b"=0.0}, "calibr coef ch 7"={"a"=1.0, "b"=0.0}}, "BGO marker\nduration[ns] 5"=0.0, "diff const [ns] 5"=0.0}  # 5172
          w21 = T9 {"5170R 0"={"Chans enable"={"Chan 0"=TRUE, "Chan 1"=TRUE, "Chan 2"=TRUE, "Chan 3"=TRUE, "Chan 4"=TRUE, "Chan 5"=TRUE, "Chan 6"=TRUE, "Chan 7"=TRUE}, "Trapez config"={"k [ns] "=1100, "m [ns] "=200, "t_decay [ns]  "=65000, "Get energy at %\n of flat top"=70}, "Trigger Cluster"={"trig config 0"={"level (V)"=-0.01, "hysteresis (V)"=0.001, "trigger slope"=enum."Negative"}, "trig config 1"={"level (V)"=-0.01, "hysteresis (V)"=0.001, "trigger slope"=enum."Negative"}, "trig config 2"={"level (V)"=-0.01, "hysteresis (V)"=0.001, "trigger slope"=enum."Negative"}, "trig config 3"={"level (V)"=-0.01, "hysteresis (V)"=0.001, "trigger slope"=enum."Negative"}, "trig config 4"={"level (V)"=-0.01, "hysteresis (V)"=0.001, "trigger slope"=enum."Negative"}, "trig config 5"={"level (V)"=-0.01, "hysteresis (V)"=0.001, "trigger slope"=enum."Negative"}, "trig config 6"={"level (V)"=-0.01, "hysteresis (V)"=0.001, "trigger slope"=enum."Negative"}, "trig config 7"={"level (V)"=-0.01, "hysteresis (V)"=0.001, "trigger slope"=enum."Negative"}}, "Calibr coef"={"calibr coef ch 0"={"a"=1.0, "b"=0.0}, "calibr coef ch 1"={"a"=1.0, "b"=0.0}, "calibr coef ch 2"={"a"=1.0, "b"=0.0}, "calibr coef ch 3"={"a"=1.0, "b"=0.0}, "calibr coef ch 4"={"a"=1.0, "b"=0.0}, "calibr coef ch 5"={"a"=1.0, "b"=0.0}, "calibr coef ch 6"={"a"=1.0, "b"=0.0}, "calibr coef ch 7"={"a"=1.0, "b"=0.0}}, "strob duration[ns]"=0.0, "diff const [ns]"=0.0}, "5170R 1"={"Chans enable"={"Chan 0"=TRUE, "Chan 1"=TRUE, "Chan 2"=TRUE, "Chan 3"=TRUE, "Chan 4"=TRUE, "Chan 5"=TRUE, "Chan 6"=TRUE, "Chan 7"=TRUE}, "Trapez config"={"k [ns] "=1100, "m [ns] "=200, "t_decay [ns]  "=65000, "Get energy at %\n of flat top"=70}, "Trigger Cluster"={"trig config 0"={"level (V)"=-0.01, "hysteresis (V)"=0.001, "trigger slope"=enum."Negative"}, "trig config 1"={"level (V)"=-0.01, "hysteresis (V)"=0.001, "trigger slope"=enum."Negative"}, "trig config 2"={"level (V)"=-0.01, "hysteresis (V)"=0.001, "trigger slope"=enum."Negative"}, "trig config 3"={"level (V)"=-0.01, "hysteresis (V)"=0.001, "trigger slope"=enum."Negative"}, "trig config 4"={"level (V)"=-0.01, "hysteresis (V)"=0.001, "trigger slope"=enum."Negative"}, "trig config 5"={"level (V)"=-0.01, "hysteresis (V)"=0.001, "trigger slope"=enum."Negative"}, "trig config 6"={"level (V)"=-0.01, "hysteresis (V)"=0.001, "trigger slope"=enum."Negative"}, "trig config 7"={"level (V)"=-0.01, "hysteresis (V)"=0.001, "trigger slope"=enum."Negative"}}, "Calibr coef"={"calibr coef ch 0"={"a"=1.0, "b"=0.0}, "calibr coef ch 1"={"a"=1.0, "b"=0.0}, "calibr coef ch 2"={"a"=1.0, "b"=0.0}, "calibr coef ch 3"={"a"=1.0, "b"=0.0}, "calibr coef ch 4"={"a"=1.0, "b"=0.0}, "calibr coef ch 5"={"a"=1.0, "b"=0.0}, "calibr coef ch 6"={"a"=1.0, "b"=0.0}, "calibr coef ch 7"={"a"=1.0, "b"=0.0}}, "strob duration[ns]"=0.0, "diff const [ns]"=0.0}, "5170R 2"={"Chans enable"={"Chan 0"=TRUE, "Chan 1"=TRUE, "Chan 2"=TRUE, "Chan 3"=TRUE, "Chan 4"=TRUE, "Chan 5"=TRUE, "Chan 6"=TRUE, "Chan 7"=TRUE}, "Trapez config"={"k [ns] "=1100, "m [ns] "=200, "t_decay [ns]  "=65000, "Get energy at %\n of flat top"=70}, "Trigger Cluster"={"trig config 0"={"level (V)"=-0.01, "hysteresis (V)"=0.001, "trigger slope"=enum."Negative"}, "trig config 1"={"level (V)"=-0.01, "hysteresis (V)"=0.001, "trigger slope"=enum."Negative"}, "trig config 2"={"level (V)"=-0.01, "hysteresis (V)"=0.001, "trigger slope"=enum."Negative"}, "trig config 3"={"level (V)"=-0.01, "hysteresis (V)"=0.001, "trigger slope"=enum."Negative"}, "trig config 4"={"level (V)"=-0.01, "hysteresis (V)"=0.001, "trigger slope"=enum."Negative"}, "trig config 5"={"level (V)"=-0.01, "hysteresis (V)"=0.001, "trigger slope"=enum."Negative"}, "trig config 6"={"level (V)"=-0.01, "hysteresis (V)"=0.001, "trigger slope"=enum."Negative"}, "trig config 7"={"level (V)"=-0.01, "hysteresis (V)"=0.001, "trigger slope"=enum."Negative"}}, "Calibr coef"={"calibr coef ch 0"={"a"=1.0, "b"=0.0}, "calibr coef ch 1"={"a"=1.0, "b"=0.0}, "calibr coef ch 2"={"a"=1.0, "b"=0.0}, "calibr coef ch 3"={"a"=1.0, "b"=0.0}, "calibr coef ch 4"={"a"=1.0, "b"=0.0}, "calibr coef ch 5"={"a"=1.0, "b"=0.0}, "calibr coef ch 6"={"a"=1.0, "b"=0.0}, "calibr coef ch 7"={"a"=1.0, "b"=0.0}}, "strob duration[ns]"=0.0, "diff const [ns]"=0.0}, "5170R 3"={"Chans enable"={"Chan 0"=TRUE, "Chan 1"=TRUE, "Chan 2"=TRUE, "Chan 3"=TRUE, "Chan 4"=TRUE, "Chan 5"=TRUE, "Chan 6"=TRUE, "Chan 7"=TRUE}, "Trapez config"={"k [ns] "=1100, "m [ns] "=200, "t_decay [ns]  "=65000, "Get energy at %\n of flat top"=70}, "Trigger Cluster"={"trig config 0"={"level (V)"=-0.01, "hysteresis (V)"=0.001, "trigger slope"=enum."Negative"}, "trig config 1"={"level (V)"=-0.01, "hysteresis (V)"=0.001, "trigger slope"=enum."Negative"}, "trig config 2"={"level (V)"=-0.01, "hysteresis (V)"=0.001, "trigger slope"=enum."Negative"}, "trig config 3"={"level (V)"=-0.01, "hysteresis (V)"=0.001, "trigger slope"=enum."Negative"}, "trig config 4"={"level (V)"=-0.01, "hysteresis (V)"=0.001, "trigger slope"=enum."Negative"}, "trig config 5"={"level (V)"=-0.01, "hysteresis (V)"=0.001, "trigger slope"=enum."Negative"}, "trig config 6"={"level (V)"=-0.01, "hysteresis (V)"=0.001, "trigger slope"=enum."Negative"}, "trig config 7"={"level (V)"=-0.01, "hysteresis (V)"=0.001, "trigger slope"=enum."Negative"}}, "Calibr coef"={"calibr coef ch 0"={"a"=1.0, "b"=0.0}, "calibr coef ch 1"={"a"=1.0, "b"=0.0}, "calibr coef ch 2"={"a"=1.0, "b"=0.0}, "calibr coef ch 3"={"a"=1.0, "b"=0.0}, "calibr coef ch 4"={"a"=1.0, "b"=0.0}, "calibr coef ch 5"={"a"=1.0, "b"=0.0}, "calibr coef ch 6"={"a"=1.0, "b"=0.0}, "calibr coef ch 7"={"a"=1.0, "b"=0.0}}, "strob duration[ns]"=0.0, "diff const [ns]"=0.0}, "5172"={"Chans enable 5"={"Chan 0"=TRUE, "Chan 1"=TRUE, "Chan 2"=TRUE, "Chan 3"=TRUE, "Chan 4"=TRUE, "Chan 5"=TRUE, "Chan 6"=TRUE, "Chan 7"=TRUE}, "Trapez config 5"={"k [ns] "=1100, "m [ns] "=200, "t_decay [ns]  "=65000, "Get energy at %\n of flat top"=70}, "Trigger Cluster 5"={"trig config 0"={"level (V)"=-0.01, "hysteresis (V)"=0.001, "trigger slope"=enum."Negative"}, "trig config 1"={"level (V)"=-0.01, "hysteresis (V)"=0.001, "trigger slope"=enum."Negative"}, "trig config 2"={"level (V)"=-0.01, "hysteresis (V)"=0.001, "trigger slope"=enum."Negative"}, "trig config 3"={"level (V)"=-0.01, "hysteresis (V)"=0.001, "trigger slope"=enum."Negative"}, "trig config 4"={"level (V)"=-0.01, "hysteresis (V)"=0.001, "trigger slope"=enum."Negative"}, "trig config 5"={"level (V)"=-0.01, "hysteresis (V)"=0.001, "trigger slope"=enum."Negative"}, "trig config 6"={"level (V)"=-0.01, "hysteresis (V)"=0.001, "trigger slope"=enum."Negative"}, "trig config 7"={"level (V)"=-0.01, "hysteresis (V)"=0.001, "trigger slope"=enum."Negative"}}, "Calibr coef 5"={"calibr coef ch 0"={"a"=1.0, "b"=0.0}, "calibr coef ch 1"={"a"=1.0, "b"=0.0}, "calibr coef ch 2"={"a"=1.0, "b"=0.0}, "calibr coef ch 3"={"a"=1.0, "b"=0.0}, "calibr coef ch 4"={"a"=1.0, "b"=0.0}, "calibr coef ch 5"={"a"=1.0, "b"=0.0}, "calibr coef ch 6"={"a"=1.0, "b"=0.0}, "calibr coef ch 7"={"a"=1.0, "b"=0.0}}, "BGO marker\nduration[ns] 5"=0.0, "diff const [ns] 5"=0.0}, "5764"={"trig marker"={"level (V)"=-0.01, "hysteresis (V)"=0.001, "trigger slope"=enum."Negative"}, "trig cfd"={"level (V)"=-0.01, "hysteresis (V)"=0.001, "trigger slope"=enum."Negative"}, "f"=0.0, "shift marker"=0.0, "marker duration"=0.0, "TAC delay"=0.0}}  # Chassi 0
          w42 = T10 {"Chans enable"={"Chan 0"=TRUE, "Chan 1"=TRUE, "Chan 2"=TRUE, "Chan 3"=TRUE, "Chan 4"=TRUE, "Chan 5"=TRUE, "Chan 6"=TRUE, "Chan 7"=TRUE}, "Trapez config"={"k [ns] "=1100, "m [ns] "=200, "t_decay [ns]  "=65000, "Get energy at %\n of flat top"=70}, "Trigger Cluster"={"trig config 0"={"level (V)"=-0.01, "hysteresis (V)"=0.001, "trigger slope"=enum."Negative"}, "trig config 1"={"level (V)"=-0.01, "hysteresis (V)"=0.001, "trigger slope"=enum."Negative"}, "trig config 2"={"level (V)"=-0.01, "hysteresis (V)"=0.001, "trigger slope"=enum."Negative"}, "trig config 3"={"level (V)"=-0.01, "hysteresis (V)"=0.001, "trigger slope"=enum."Negative"}, "trig config 4"={"level (V)"=-0.01, "hysteresis (V)"=0.001, "trigger slope"=enum."Negative"}, "trig config 5"={"level (V)"=-0.01, "hysteresis (V)"=0.001, "trigger slope"=enum."Negative"}, "trig config 6"={"level (V)"=-0.01, "hysteresis (V)"=0.001, "trigger slope"=enum."Negative"}, "trig config 7"={"level (V)"=-0.01, "hysteresis (V)"=0.001, "trigger slope"=enum."Negative"}}, "Calibr coef"={"calibr coef ch 0"={"a"=1.0, "b"=0.0}, "calibr coef ch 1"={"a"=1.0, "b"=0.0}, "calibr coef ch 2"={"a"=1.0, "b"=0.0}, "calibr coef ch 3"={"a"=1.0, "b"=0.0}, "calibr coef ch 4"={"a"=1.0, "b"=0.0}, "calibr coef ch 5"={"a"=1.0, "b"=0.0}, "calibr coef ch 6"={"a"=1.0, "b"=0.0}, "calibr coef ch 7"={"a"=1.0, "b"=0.0}}, "strob duration[ns]"=0.0, "diff const [ns]"=0.0}  # 5170R
          w14 = T11 {"Chassi 0"={"5170R 0"={"Chans enable"={"Chan 0"=TRUE, "Chan 1"=TRUE, "Chan 2"=TRUE, "Chan 3"=TRUE, "Chan 4"=TRUE, "Chan 5"=TRUE, "Chan 6"=TRUE, "Chan 7"=TRUE}, "Trapez config"={"k [ns] "=1100, "m [ns] "=200, "t_decay [ns]  "=65000, "Get energy at %\n of flat top"=70}, "Trigger Cluster"={"trig config 0"={"level (V)"=-0.01, "hysteresis (V)"=0.001, "trigger slope"=enum."Negative"}, "trig config 1"={"level (V)"=-0.01, "hysteresis (V)"=0.001, "trigger slope"=enum."Negative"}, "trig config 2"={"level (V)"=-0.01, "hysteresis (V)"=0.001, "trigger slope"=enum."Negative"}, "trig config 3"={"level (V)"=-0.01, "hysteresis (V)"=0.001, "trigger slope"=enum."Negative"}, "trig config 4"={"level (V)"=-0.01, "hysteresis (V)"=0.001, "trigger slope"=enum."Negative"}, "trig config 5"={"level (V)"=-0.01, "hysteresis (V)"=0.001, "trigger slope"=enum."Negative"}, "trig config 6"={"level (V)"=-0.01, "hysteresis (V)"=0.001, "trigger slope"=enum."Negative"}, "trig config 7"={"level (V)"=-0.01, "hysteresis (V)"=0.001, "trigger slope"=enum."Negative"}}, "Calibr coef"={"calibr coef ch 0"={"a"=1.0, "b"=0.0}, "calibr coef ch 1"={"a"=1.0, "b"=0.0}, "calibr coef ch 2"={"a"=1.0, "b"=0.0}, "calibr coef ch 3"={"a"=1.0, "b"=0.0}, "calibr coef ch 4"={"a"=1.0, "b"=0.0}, "calibr coef ch 5"={"a"=1.0, "b"=0.0}, "calibr coef ch 6"={"a"=1.0, "b"=0.0}, "calibr coef ch 7"={"a"=1.0, "b"=0.0}}, "strob duration[ns]"=0.0, "diff const [ns]"=0.0}, "5170R 1"={"Chans enable"={"Chan 0"=TRUE, "Chan 1"=TRUE, "Chan 2"=TRUE, "Chan 3"=TRUE, "Chan 4"=TRUE, "Chan 5"=TRUE, "Chan 6"=TRUE, "Chan 7"=TRUE}, "Trapez config"={"k [ns] "=1100, "m [ns] "=200, "t_decay [ns]  "=65000, "Get energy at %\n of flat top"=70}, "Trigger Cluster"={"trig config 0"={"level (V)"=-0.01, "hysteresis (V)"=0.001, "trigger slope"=enum."Negative"}, "trig config 1"={"level (V)"=-0.01, "hysteresis (V)"=0.001, "trigger slope"=enum."Negative"}, "trig config 2"={"level (V)"=-0.01, "hysteresis (V)"=0.001, "trigger slope"=enum."Negative"}, "trig config 3"={"level (V)"=-0.01, "hysteresis (V)"=0.001, "trigger slope"=enum."Negative"}, "trig config 4"={"level (V)"=-0.01, "hysteresis (V)"=0.001, "trigger slope"=enum."Negative"}, "trig config 5"={"level (V)"=-0.01, "hysteresis (V)"=0.001, "trigger slope"=enum."Negative"}, "trig config 6"={"level (V)"=-0.01, "hysteresis (V)"=0.001, "trigger slope"=enum."Negative"}, "trig config 7"={"level (V)"=-0.01, "hysteresis (V)"=0.001, "trigger slope"=enum."Negative"}}, "Calibr coef"={"calibr coef ch 0"={"a"=1.0, "b"=0.0}, "calibr coef ch 1"={"a"=1.0, "b"=0.0}, "calibr coef ch 2"={"a"=1.0, "b"=0.0}, "calibr coef ch 3"={"a"=1.0, "b"=0.0}, "calibr coef ch 4"={"a"=1.0, "b"=0.0}, "calibr coef ch 5"={"a"=1.0, "b"=0.0}, "calibr coef ch 6"={"a"=1.0, "b"=0.0}, "calibr coef ch 7"={"a"=1.0, "b"=0.0}}, "strob duration[ns]"=0.0, "diff const [ns]"=0.0}, "5170R 2"={"Chans enable"={"Chan 0"=TRUE, "Chan 1"=TRUE, "Chan 2"=TRUE, "Chan 3"=TRUE, "Chan 4"=TRUE, "Chan 5"=TRUE, "Chan 6"=TRUE, "Chan 7"=TRUE}, "Trapez config"={"k [ns] "=1100, "m [ns] "=200, "t_decay [ns]  "=65000, "Get energy at %\n of flat top"=70}, "Trigger Cluster"={"trig config 0"={"level (V)"=-0.01, "hysteresis (V)"=0.001, "trigger slope"=enum."Negative"}, "trig config 1"={"level (V)"=-0.01, "hysteresis (V)"=0.001, "trigger slope"=enum."Negative"}, "trig config 2"={"level (V)"=-0.01, "hysteresis (V)"=0.001, "trigger slope"=enum."Negative"}, "trig config 3"={"level (V)"=-0.01, "hysteresis (V)"=0.001, "trigger slope"=enum."Negative"}, "trig config 4"={"level (V)"=-0.01, "hysteresis (V)"=0.001, "trigger slope"=enum."Negative"}, "trig config 5"={"level (V)"=-0.01, "hysteresis (V)"=0.001, "trigger slope"=enum."Negative"}, "trig config 6"={"level (V)"=-0.01, "hysteresis (V)"=0.001, "trigger slope"=enum."Negative"}, "trig config 7"={"level (V)"=-0.01, "hysteresis (V)"=0.001, "trigger slope"=enum."Negative"}}, "Calibr coef"={"calibr coef ch 0"={"a"=1.0, "b"=0.0}, "calibr coef ch 1"={"a"=1.0, "b"=0.0}, "calibr coef ch 2"={"a"=1.0, "b"=0.0}, "calibr coef ch 3"={"a"=1.0, "b"=0.0}, "calibr coef ch 4"={"a"=1.0, "b"=0.0}, "calibr coef ch 5"={"a"=1.0, "b"=0.0}, "calibr coef ch 6"={"a"=1.0, "b"=0.0}, "calibr coef ch 7"={"a"=1.0, "b"=0.0}}, "strob duration[ns]"=0.0, "diff const [ns]"=0.0}, "5170R 3"={"Chans enable"={"Chan 0"=TRUE, "Chan 1"=TRUE, "Chan 2"=TRUE, "Chan 3"=TRUE, "Chan 4"=TRUE, "Chan 5"=TRUE, "Chan 6"=TRUE, "Chan 7"=TRUE}, "Trapez config"={"k [ns] "=1100, "m [ns] "=200, "t_decay [ns]  "=65000, "Get energy at %\n of flat top"=70}, "Trigger Cluster"={"trig config 0"={"level (V)"=-0.01, "hysteresis (V)"=0.001, "trigger slope"=enum."Negative"}, "trig config 1"={"level (V)"=-0.01, "hysteresis (V)"=0.001, "trigger slope"=enum."Negative"}, "trig config 2"={"level (V)"=-0.01, "hysteresis (V)"=0.001, "trigger slope"=enum."Negative"}, "trig config 3"={"level (V)"=-0.01, "hysteresis (V)"=0.001, "trigger slope"=enum."Negative"}, "trig config 4"={"level (V)"=-0.01, "hysteresis (V)"=0.001, "trigger slope"=enum."Negative"}, "trig config 5"={"level (V)"=-0.01, "hysteresis (V)"=0.001, "trigger slope"=enum."Negative"}, "trig config 6"={"level (V)"=-0.01, "hysteresis (V)"=0.001, "trigger slope"=enum."Negative"}, "trig config 7"={"level (V)"=-0.01, "hysteresis (V)"=0.001, "trigger slope"=enum."Negative"}}, "Calibr coef"={"calibr coef ch 0"={"a"=1.0, "b"=0.0}, "calibr coef ch 1"={"a"=1.0, "b"=0.0}, "calibr coef ch 2"={"a"=1.0, "b"=0.0}, "calibr coef ch 3"={"a"=1.0, "b"=0.0}, "calibr coef ch 4"={"a"=1.0, "b"=0.0}, "calibr coef ch 5"={"a"=1.0, "b"=0.0}, "calibr coef ch 6"={"a"=1.0, "b"=0.0}, "calibr coef ch 7"={"a"=1.0, "b"=0.0}}, "strob duration[ns]"=0.0, "diff const [ns]"=0.0}, "5172"={"Chans enable 5"={"Chan 0"=TRUE, "Chan 1"=TRUE, "Chan 2"=TRUE, "Chan 3"=TRUE, "Chan 4"=TRUE, "Chan 5"=TRUE, "Chan 6"=TRUE, "Chan 7"=TRUE}, "Trapez config 5"={"k [ns] "=1100, "m [ns] "=200, "t_decay [ns]  "=65000, "Get energy at %\n of flat top"=70}, "Trigger Cluster 5"={"trig config 0"={"level (V)"=-0.01, "hysteresis (V)"=0.001, "trigger slope"=enum."Negative"}, "trig config 1"={"level (V)"=-0.01, "hysteresis (V)"=0.001, "trigger slope"=enum."Negative"}, "trig config 2"={"level (V)"=-0.01, "hysteresis (V)"=0.001, "trigger slope"=enum."Negative"}, "trig config 3"={"level (V)"=-0.01, "hysteresis (V)"=0.001, "trigger slope"=enum."Negative"}, "trig config 4"={"level (V)"=-0.01, "hysteresis (V)"=0.001, "trigger slope"=enum."Negative"}, "trig config 5"={"level (V)"=-0.01, "hysteresis (V)"=0.001, "trigger slope"=enum."Negative"}, "trig config 6"={"level (V)"=-0.01, "hysteresis (V)"=0.001, "trigger slope"=enum."Negative"}, "trig config 7"={"level (V)"=-0.01, "hysteresis (V)"=0.001, "trigger slope"=enum."Negative"}}, "Calibr coef 5"={"calibr coef ch 0"={"a"=1.0, "b"=0.0}, "calibr coef ch 1"={"a"=1.0, "b"=0.0}, "calibr coef ch 2"={"a"=1.0, "b"=0.0}, "calibr coef ch 3"={"a"=1.0, "b"=0.0}, "calibr coef ch 4"={"a"=1.0, "b"=0.0}, "calibr coef ch 5"={"a"=1.0, "b"=0.0}, "calibr coef ch 6"={"a"=1.0, "b"=0.0}, "calibr coef ch 7"={"a"=1.0, "b"=0.0}}, "BGO marker\nduration[ns] 5"=0.0, "diff const [ns] 5"=0.0}, "5764"={"trig marker"={"level (V)"=-0.01, "hysteresis (V)"=0.001, "trigger slope"=enum."Negative"}, "trig cfd"={"level (V)"=-0.01, "hysteresis (V)"=0.001, "trigger slope"=enum."Negative"}, "f"=0.0, "shift marker"=0.0, "marker duration"=0.0, "TAC delay"=0.0}}}  # System
          # "5764"
          # "5172"
          # "5170R"
          # "5170R"
          # "5170R"
          # "5170R"
          # "5170R: 1 - channel enable, 2 - trigger configs, 3 - calibration coeffs, 4 - trapeze configs, 5 - strob duration, 6 - diff const\n5172:   1 - channel enable, 2 - trigger configs, 3 - calibration coeffs, 4 - trapeze configs, 5 - BGO marker duration, 6 - diff const\n5764:   1 - marker trig configs, 2 - cfd trigger configs, 3 - f, 4 - marker shift, 5 - marker duration, 6 - TAC delay"
          n3 = Concatenate Strings("file name", ".xml" ("string")) -> (w5:string)
          n4 = String To Path(string=w5) -> (path=w4:path)
          n5 = Build Path(base path="folder", name or relative path=w4) -> (appended path=w10:path)
          n6 = Bundle By Name(cluster=w35, "Chans enable 5"="Chans enable 5", "Trigger Cluster 5"="Trigger Cluster 5", "Calibr coef 5"="Calibr coef 5", "Trapez config 5"="Trapez config 5", "BGO marker\nduration[ns] 5"="BGO marker\nduration[ns] 5", "diff const [ns] 5"="diff const [ns] 5") -> (w16:T8)
          n7 = Bundle By Name(cluster=w42, "Chans enable"="Chans enable", "Trigger Cluster"="Trigger Cluster", "Calibr coef"="Calibr coef", "Trapez config"="Trapez config", "strob duration[ns]"="strob duration[ns]", "diff const [ns]"="diff const [ns]") -> (w20:T10)
          n8 = Bundle By Name(cluster=w42, "Chans enable"="Chans enable 2", "Trigger Cluster"="Trigger Cluster 2", "Calibr coef"="Calibr coef 2", "Trapez config"="Trapez config 2", "strob duration[ns]"="strob duration[ns] 2", "diff const [ns]"="diff const [ns] 2") -> (w19:T10)
          n9 = Bundle By Name(cluster=w42, "Chans enable"="Chans enable 3", "Trigger Cluster"="Trigger Cluster 3", "Calibr coef"="Calibr coef 3", "Trapez config"="Trapez config 3", "strob duration[ns]"="strob duration[ns] 3", "diff const [ns]"="diff const [ns] 3") -> (w18:T10)
          n10 = Bundle By Name(cluster=w42, "Chans enable"="Chans enable 4", "Trigger Cluster"="Trigger Cluster 4", "Calibr coef"="Calibr coef 4", "Trapez config"="Trapez config 4", "strob duration[ns]"="strob duration[ns] 4", "diff const [ns]"="diff const [ns] 4") -> (w17:T10)
          n11 = Bundle By Name(cluster=w28, "trig marker"="trig marker", "trig cfd"="trig cfd", "f"="f", "shift marker"="shift marker", "marker duration"="marker duration", "TAC delay"="TAC delay") -> (w15:T7)
          n12 = local write "Writing done successfully"(FALSE ("Writing done successfully")) -> ()
          n13 = Bundle By Name(cluster=w21, "5170R 0"=w20, "5170R 1"=w19, "5170R 2"=w18, "5170R 3"=w17, "5172"=w16, "5764"=w15) -> (w13:T9)
          n14 = Bundle By Name(cluster=w14, "Chassi 0"=w13) -> (w12:T11)
          n15 = Flatten To XML(6:w12) -> (2:w9:string)
          n16 = call-poly <vilib>:"Write to XML File.vi"("XML Input"=w9, "XML File Path"=w10) -> ("error out"=w8:errorcluster)  [unwired: 7 in, 2 out]
        }
        frame #1 {
          n17 = Unbundle By Name(w63) -> ("status"=w62:bool)
          n18 = Not(x=w62) -> (.not. x?=→"Writing done successfully":bool)
        }
      }
    }
    frame "Set common configs" {
      w75 = T6 {"calibr coef ch 0"={"a"=1.0, "b"=0.0}, "calibr coef ch 1"={"a"=1.0, "b"=0.0}, "calibr coef ch 2"={"a"=1.0, "b"=0.0}, "calibr coef ch 3"={"a"=1.0, "b"=0.0}, "calibr coef ch 4"={"a"=1.0, "b"=0.0}, "calibr coef ch 5"={"a"=1.0, "b"=0.0}, "calibr coef ch 6"={"a"=1.0, "b"=0.0}, "calibr coef ch 7"={"a"=1.0, "b"=0.0}} ("Calibr coef")
      n19 = local write "Writing done successfully"(FALSE ("Writing done successfully")) -> ()
      n20 = local write "Calibr coef"(w75) -> ()
      n21 = local write "Calibr coef 2"(w75) -> ()
      n22 = local write "Calibr coef 3"(w75) -> ()
      n23 = local write "Calibr coef 4"(w75) -> ()
      n24 = local write "Calibr coef 5"(w75) -> ()
      n25 = local write "Chans enable"("Chans enable 6") -> ()
      n26 = local write "Chans enable 2"("Chans enable 6") -> ()
      n27 = local write "Chans enable 3"("Chans enable 6") -> ()
      n28 = local write "Chans enable 4"("Chans enable 6") -> ()
      n29 = local write "Chans enable 5"("Chans enable 6") -> ()
      n30 = local write "Trapez config"("Trapez config 6") -> ()
      n31 = local write "Trapez config 2"("Trapez config 6") -> ()
      n32 = local write "Trapez config 3"("Trapez config 6") -> ()
      n33 = local write "Trapez config 4"("Trapez config 6") -> ()
      n34 = local write "Trapez config 5"("Trapez config 6") -> ()
      n35 = local write "strob duration[ns]"("strob duration[ns] 5") -> ()
      n36 = local write "strob duration[ns] 2"("strob duration[ns] 5") -> ()
      n37 = local write "strob duration[ns] 3"("strob duration[ns] 5") -> ()
      n38 = local write "strob duration[ns] 4"("strob duration[ns] 5") -> ()
      n39 = local write "strob duration[ns] 5"("strob duration[ns] 5") -> ()
      n40 = local write "diff const [ns]"("diff const [ns] 6") -> ()
      n41 = local write "diff const [ns] 2"("diff const [ns] 6") -> ()
      n42 = local write "diff const [ns] 3"("diff const [ns] 6") -> ()
      n43 = local write "diff const [ns] 4"("diff const [ns] 6") -> ()
      n44 = local write "diff const [ns] 5"("diff const [ns] 6") -> ()
      n45 = Bundle("common trig 5170R 0-1"="common trig 5170R 0-1", "common trig 5170R 0-1"="common trig 5170R 0-1", "common trig 5170R 0-1"="common trig 5170R 0-1", "common trig 5170R 0-1"="common trig 5170R 0-1", "common trig 5170R 0-1"="common trig 5170R 0-1", "common trig 5170R 0-1"="common trig 5170R 0-1", "common trig 5170R 0-1"="common trig 5170R 0-1", "common trig 5170R 0-1"="common trig 5170R 0-1") -> (w71:T12)  [unwired: 1 in]
      n46 = Bundle("common trig 5170R 2-3"="common trig 5170R 2-3", "common trig 5170R 2-3"="common trig 5170R 2-3", "common trig 5170R 2-3"="common trig 5170R 2-3", "common trig 5170R 2-3"="common trig 5170R 2-3", "common trig 5170R 2-3"="common trig 5170R 2-3", "common trig 5170R 2-3"="common trig 5170R 2-3", "common trig 5170R 2-3"="common trig 5170R 2-3", "common trig 5170R 2-3"="common trig 5170R 2-3") -> (w69:T13)  [unwired: 1 in]
      n47 = Bundle("common trig 5172"="common trig 5172", "common trig 5172"="common trig 5172", "common trig 5172"="common trig 5172", "common trig 5172"="common trig 5172", "common trig 5172"="common trig 5172", "common trig 5172"="common trig 5172", "common trig 5172"="common trig 5172", "common trig 5172"="common trig 5172") -> (w67:T14)  [unwired: 1 in]
      n48 = local write "Trigger Cluster"(w71) -> ()
      n49 = local write "Trigger Cluster 2"(w71) -> ()
      n50 = local write "Trigger Cluster 3"(w69) -> ()
      n51 = local write "Trigger Cluster 4"(w69) -> ()
      n52 = local write "Trigger Cluster 5"(w67) -> ()
      n53 = disable-structure shown="Disabled" {
        frame Disabled {
          n54 = local read item#-1() -> ()  [unwired: 1 in]
          n55 = local read item#-1() -> ()  [unwired: 1 in]
          n56 = local read item#-1() -> ()  [unwired: 1 in]
          n57 = local read item#-1() -> ()  [unwired: 1 in]
          n58 = local read item#-1() -> ()  [unwired: 1 in]
          n59 = local read item#-1() -> ()  [unwired: 1 in]
          n60 = local read item#-1() -> ()  [unwired: 1 in]
          n61 = local read item#-1() -> ()  [unwired: 1 in]
          n62 = local read item#-1() -> ()  [unwired: 1 in]
          n63 = local read item#-1() -> ()  [unwired: 1 in]
          n64 = local read item#-1() -> ()  [unwired: 1 in]
          n65 = local read item#-1() -> ()  [unwired: 1 in]
          n66 = local read item#-1() -> ()  [unwired: 1 in]
          n67 = local read item#-1() -> ()  [unwired: 1 in]
          n68 = local read item#-1() -> ()  [unwired: 1 in]
          n69 = local read item#-1() -> ()  [unwired: 1 in]
          n70 = local read item#-1() -> ()  [unwired: 1 in]
          n71 = local read item#-1() -> ()  [unwired: 1 in]
          n72 = local read item#-1() -> ()  [unwired: 1 in]
          n73 = local read item#-1() -> ()  [unwired: 1 in]
          n74 = local read item#-1() -> ()  [unwired: 1 in]
          n75 = local read item#-1() -> ()  [unwired: 1 in]
          n76 = local read item#-1() -> ()  [unwired: 1 in]
          n77 = local read item#-1() -> ()  [unwired: 1 in]
          n78 = local read item#-1() -> ()  [unwired: 1 in]
        }
        frame Enabled {
        }
      }
    }
  }
